vi "ReconnectProcedure.vi"   [LabVIEW 2014]
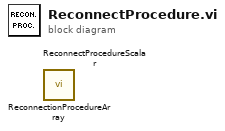
[diagram p0: block diagram]
diagram:
  n1 = call "ReconnectionProcedureArray.vi"() -> ()  [unwired: 3 in, 2 out]
  n2 = call "ReconnectProcedureScalar.vi"() -> ()  [unwired: 3 in, 2 out]
